vi "Right regions to subsectors.vi"(1 "Right Regions":bool[](array[boolean])) -> (0 "Right subsector array":bool[][](array[boolean]))   [LabVIEW 2009]
doc: "Converts the marked regions to\ntwo dimensional arrays. Each \nelement in such an array is an\narray of marked regions for a \nparticular 18 degree wedge of\nthe sick's field of view, called a\n\"subector\"."
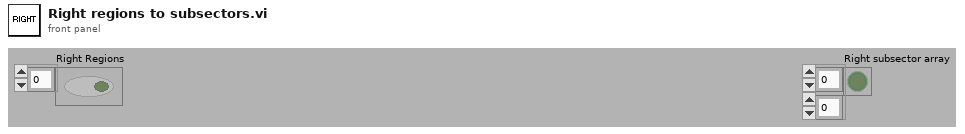
[diagram p1: front panel]
types:
  T1 = cluster{"Right Regions [0]":bool, "Right Regions [1]":bool, "Right Regions [2]":bool, "Right Regions [3]":bool, "Right Regions [4]":bool, "Right Regions [5]":bool, "Right Regions [6]":bool, "Right Regions [7]":bool, "Right Regions [8]":bool, "Right Regions [9]":bool, "Right Regions [10]":bool, "Right Regions [11]":bool, "Right Regions [12]":bool, "Right Regions [13]":bool, "Right Regions [14]":bool, "Right Regions [15]":bool, "Right Regions [16]":bool, "Right Regions [17]":bool, "Right Regions [18]":bool}
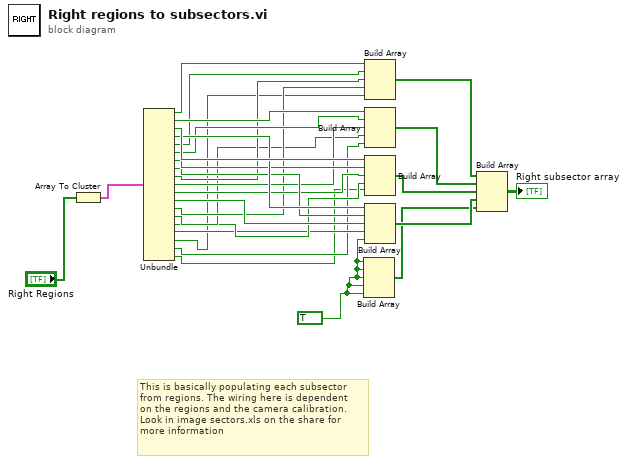
[diagram p0: block diagram]
diagram:
  w11 = TRUE
  # "This is basically populating each subsector\nfrom regions. The wiring here is dependent\non the regions and the camera calibration.\nLook in image sectors.xls on the share for\nmore information"
  n1 = Array To Cluster(array="Right Regions") -> (cluster=w28:T1)
  n2 = Unbundle(w28) -> ("Right Regions [0]"=w27:bool, "Right Regions [1]"=w26:bool, "Right Regions [2]"=w25:bool, "Right Regions [3]"=w24:bool, "Right Regions [4]"=w23:bool, "Right Regions [5]"=w22:bool, "Right Regions [6]"=w21:bool, "Right Regions [7]"=w20:bool, "Right Regions [8]"=w19:bool, "Right Regions [9]"=w18:bool, "Right Regions [10]"=w17:bool, "Right Regions [11]"=w16:bool, "Right Regions [12]"=w15:bool, "Right Regions [13]"=w14:bool, "Right Regions [14]"=w13:bool, "Right Regions [15]"=w12:bool, "Right Regions [16]"=w10:bool, "Right Regions [17]"=w9:bool, "Right Regions [18]"=w8:bool)
  n3 = Build Array(w11, w11, w11, w11, w11) -> (w3:bool[])
  n4 = Build Array(w27, w23, w19, w15, w10) -> (w7:bool[])
  n5 = Build Array(w26, w22, w18, w14, w9) -> (w6:bool[])
  n6 = Build Array(w25, w21, w17, w13, w8) -> (w5:bool[])
  n7 = Build Array(w24, w20, w16, w12, w11) -> (w4:bool[])
  n8 = Build Array(w7, w6, w5, w4, w3) -> (→"Right subsector array":bool[][])
